vi "FTW-Regex-Destroy.vi"(0 "Regex":refnum<class "FTW-Regex.lvclass">, 11 "error in":errorcluster) -> (15 "error out":errorcluster)   [LabVIEW 2014, in "FTW-Regex.lvclass"]
uses:
  FTW-Regex.lvclass
  FTW-Regex.lvclass/FTW-Regex.ctl
  error/FTW-ERR-ThrowGenericError.vi
  error/FTW-ERR-ThrowError.vi
  error/FTW-ERR-CallChain.vi
  string/FTW-STR-ReplaceWhitespace.vi
panel:
  # "Inputs"
  # "Outputs"
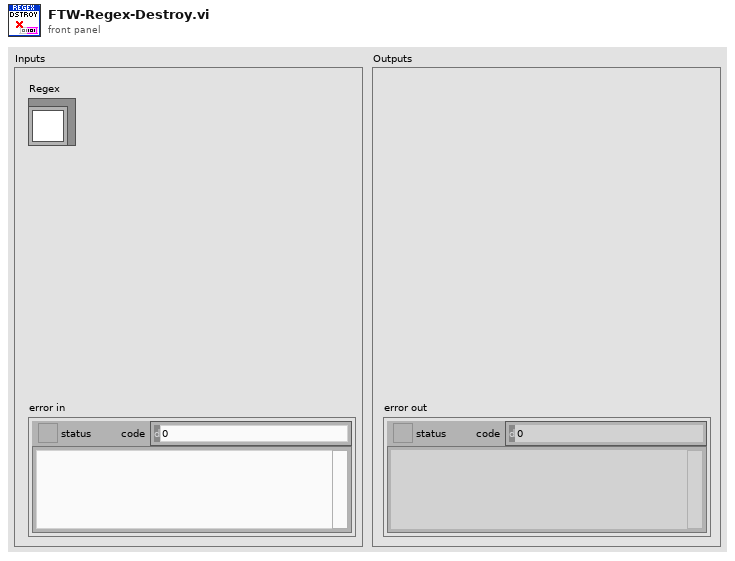
[diagram p1: front panel]
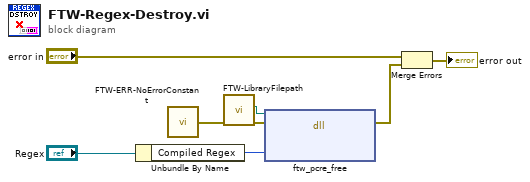
[diagram p0: block diagram]
diagram:
  n1 = Unbundle By Name("Regex") -> ("Compiled Regex"=w5:u64)
  n2 = call "FTW-ERR-NoErrorConstant.vi"() -> ("no error"=w1:errorcluster)
  n3 = call "FTW-LibraryFilepath.vi"("error in"=w1) -> ("error out"=w7:errorcluster, "Library Filepath"=w8:path)  [unwired: 8 in, 1 out]
  n4 = dll-call lib="?" fn="ftw_pcre_free"(path in=w8, error in=w7, "Compiled Regex"=w5) -> (error out=w3:errorcluster)  [unwired: 3 in, 1 out]
  n5 = Merge Errors("error in", w3) -> (→"error out":errorcluster)
